vi "Dialog_debug (SubVI).vi"() -> ()   [LabVIEW 2017]
doc: "Use this template to create a dialog box with event handling."
uses:
  Control_EU/UNDT_ClusterPackRevers (Type).ctl
  Global_SNK3_HF.vi
panel:
  in  "Tab Control":enum32{"UNDT_Cl 1", "Page 2"}(tab)
  out "UNDT_Cl0":T1={"PacketCounter"=998360, "Gain Coeff"=0.0, "SamplingInterval"=2e-08, "Lose Packet"=8, "EncodersParam2"=0, "EncodersParam1"=0, "Reserve 1"=0, "Mux TX/RX"=0, "ScanDelay"=0, "CRC 8"=86, "ScanDuration"=500, "N chanel"=0, "GlobalTime2"=63660000, "GlobalTime1"=11423, "N tick"=0, "Ncycle"=15329, "FrameFormatVersion"=1, "MagicWord"=305419896, "Overload"=FALSE} {"Gain Coeff" format="%_5e"; "Reserve 1" format="%02x"; "Mux TX/RX" format="%02x"; "ScanDelay" format="%02x"; "SamplingInterval" format="%_3e"; "Lose Packet" format="%08x"; "EncodersParam2" format="%016x"; "EncodersParam1" format="%016x"; "CRC 8" format="%02x"; "N chanel" format="%02x"; "N tick" format="%02x"; "FrameFormatVersion" format="%02x"; "MagicWord" format="%.0x"}
  out "UNDT_Cl1":T1={"PacketCounter"=998360, "Gain Coeff"=0.0, "SamplingInterval"=2e-08, "Lose Packet"=8, "EncodersParam2"=0, "EncodersParam1"=0, "Reserve 1"=0, "Mux TX/RX"=0, "ScanDelay"=0, "CRC 8"=86, "ScanDuration"=500, "N chanel"=0, "GlobalTime2"=63660000, "GlobalTime1"=11423, "N tick"=0, "Ncycle"=15329, "FrameFormatVersion"=1, "MagicWord"=305419896, "Overload"=FALSE} {"Gain Coeff" format="%_5e"; "Reserve 1" format="%02x"; "Mux TX/RX" format="%02x"; "ScanDelay" format="%02x"; "SamplingInterval" format="%_3e"; "Lose Packet" format="%08x"; "EncodersParam2" format="%016x"; "EncodersParam1" format="%016x"; "CRC 8" format="%02x"; "N chanel" format="%02x"; "N tick" format="%02x"; "FrameFormatVersion" format="%02x"; "MagicWord" format="%.0x"}
  out "UDP0_iter_count":i32=7055
  out "UDP0_timeout":i32=1000
  out "UDP0_port":u16=1555
  out "UDP0_address":u32=3232235999 format="%x"
  out "UDP0_AscanLostPack":u32
  out "UDP0_offset":i32
  out "UDP0_Reserv":u8
  out "UDP0_length":i32=2052
  out "UDP0_packet_nuber":u32=1995311
  out "UDP0_packet_size":u16=652
  out "UDP0_LostPack":u32 caption="UDP0__lost_pack"
  out "UDP0_CRC8_bad":u32
  out "UDP0_PackEnd_bad":u32
  in  "stop":bool
  out "TblParam0":sgl[][](array[numeric])
  out "TblParam1":sgl[][](array[numeric])
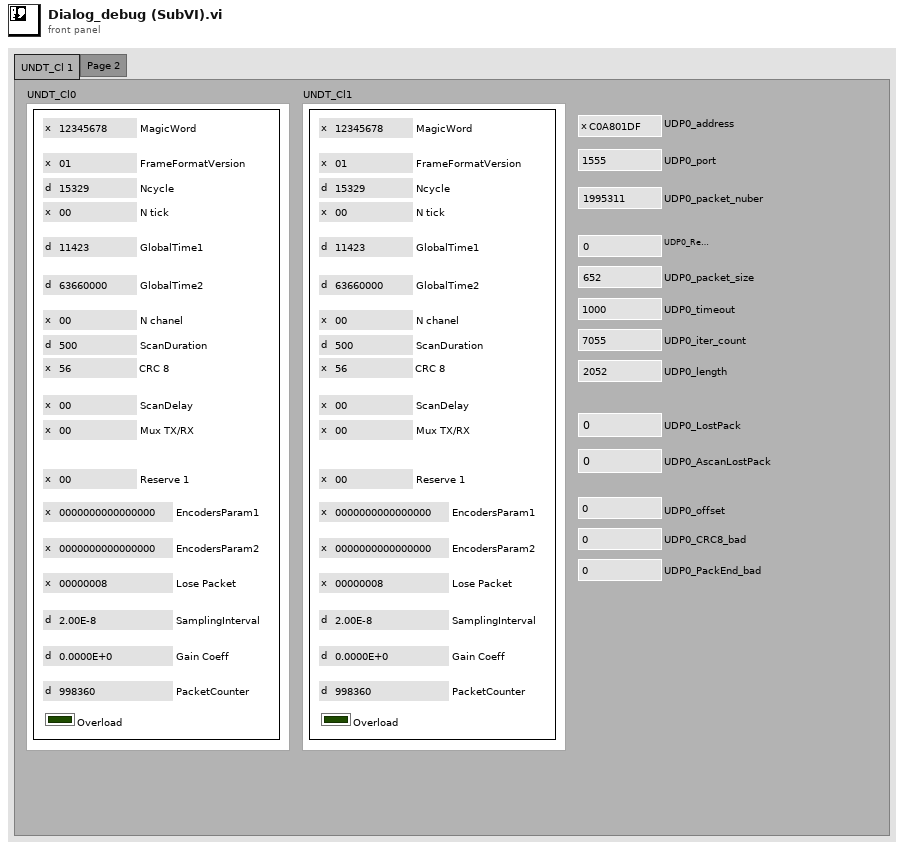
[diagram p1: front panel]
types:
  T1 = typedef "UNDT_ClusterPackRevers (Type).ctl" = cluster{"PacketCounter":u32, "Gain Coeff":sgl, "SamplingInterval":sgl, "Lose Packet":u32, "EncodersParam2":u64, "EncodersParam1":u64, "Reserve 1":u8, "Mux TX/RX":u8, "ScanDelay":u16, "CRC 8":u8, "ScanDuration":u16, "N chanel":u8, "GlobalTime2":u32, "GlobalTime1":u32, "N tick":u8, "Ncycle":u16, "FrameFormatVersion":u8, "MagicWord":u32, "Overload":bool}
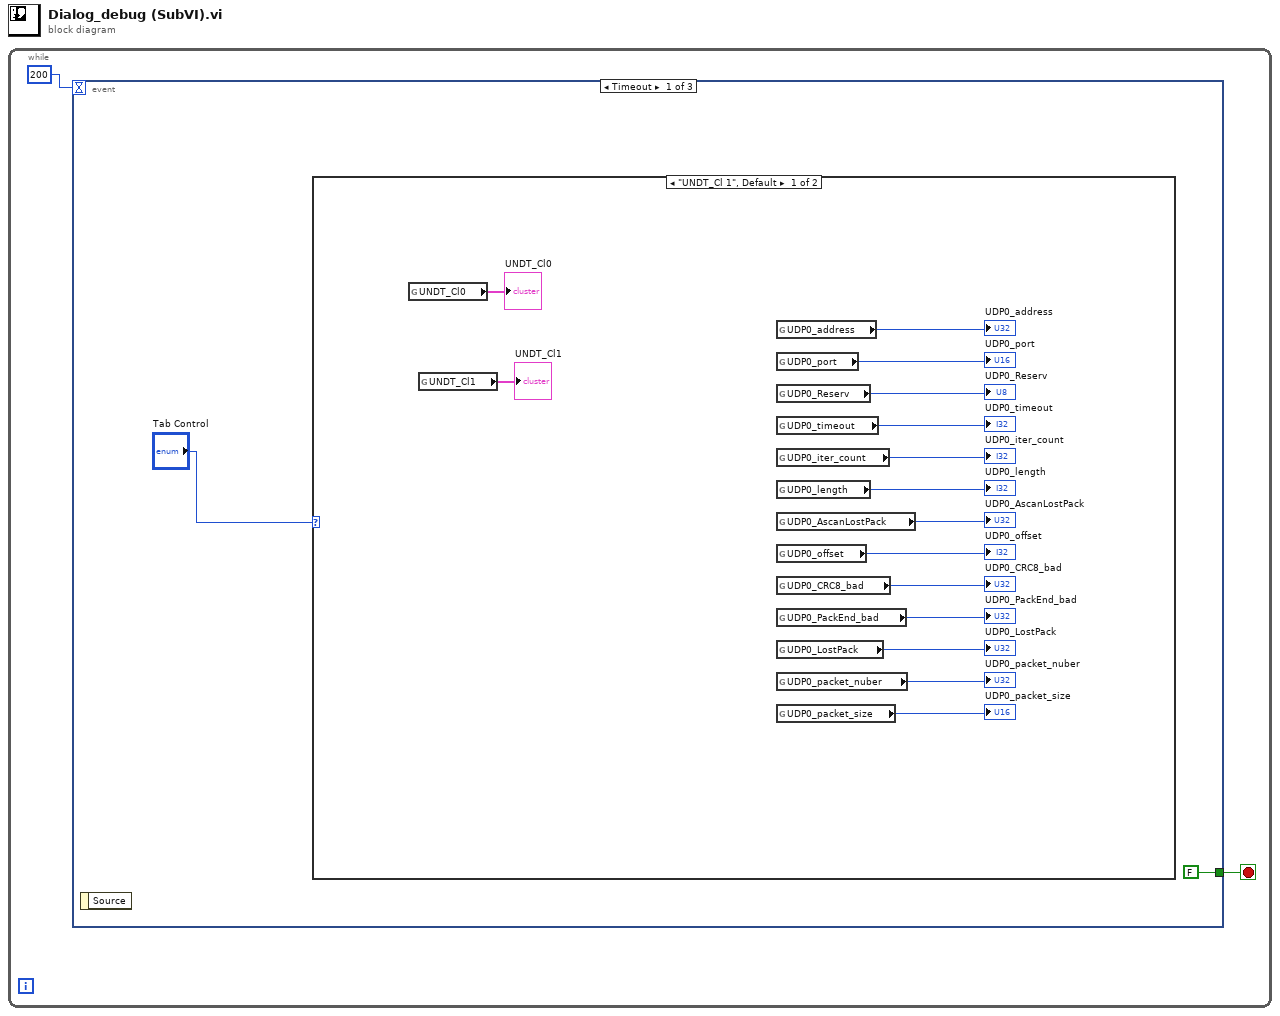
[diagram p0: block diagram]
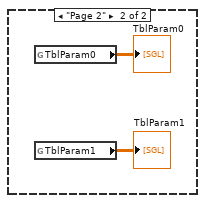
[diagram p2: hidden frame]
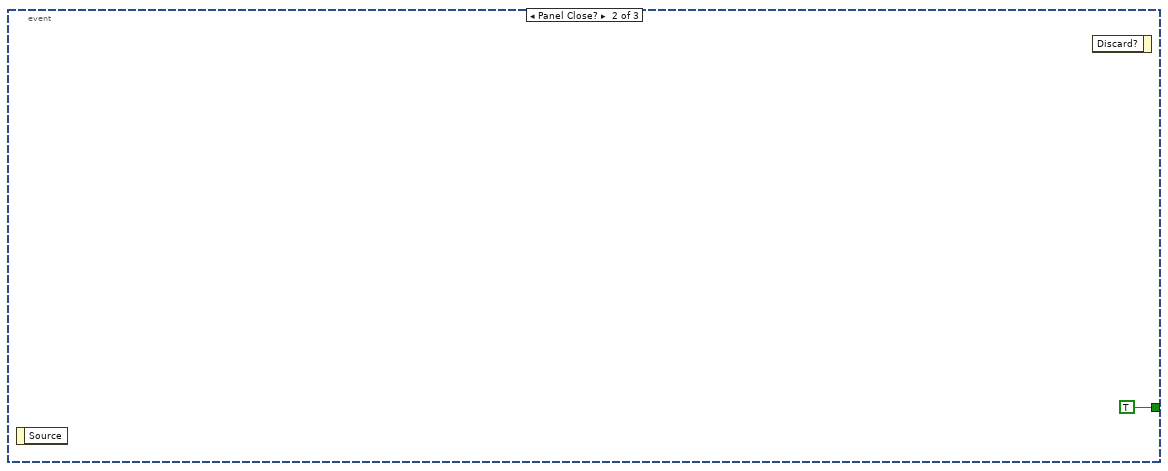
[diagram p3: hidden frame]
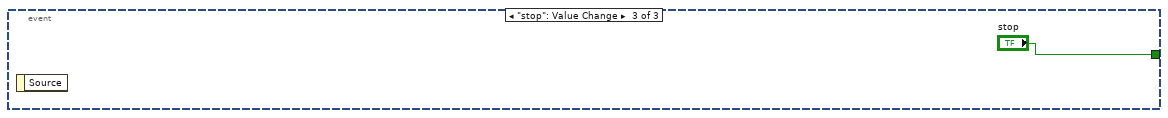
[diagram p4: hidden frame]
diagram:
  n1 = while {
    stop <- w2 stop-if-true
    n2 = event shown="[0] Timeout" {
      selector: _ -> [_ _ _]
      dyn-events: _ -> [_ _ _]
      timeout: 200 -> [_ _ _]
      tunnel: [FALSE ("stop") TRUE ("Stop?") "stop"] -> w2
      event Timeout {
        n3 = event-data() -> ()  [unwired: 1 in, 1 out]
        n4 = case shown="\"UNDT_Cl 1\", Default" "Tab Control" {
          frame "UNDT_Cl 1", Default {
            n5 = global read "Global_SNK3_HF.vi" "UNDT_Cl0"() -> (→"UNDT_Cl0":T1)
            n6 = global read "Global_SNK3_HF.vi" "UNDT_Cl1"() -> (→"UNDT_Cl1":T1)
            n7 = global read "Global_SNK3_HF.vi" "UDP0_address"() -> (→"UDP0_address":u32)
            n8 = global read "Global_SNK3_HF.vi" "UDP0_port"() -> (→"UDP0_port":u16)
            n9 = global read "Global_SNK3_HF.vi" "UDP0_Reserv"() -> (→"UDP0_Reserv":u8)
            n10 = global read "Global_SNK3_HF.vi" "UDP0_timeout"() -> (→"UDP0_timeout":i32)
            n11 = global read "Global_SNK3_HF.vi" "UDP0_iter_count"() -> (→"UDP0_iter_count":i32)
            n12 = global read "Global_SNK3_HF.vi" "UDP0_length"() -> (→"UDP0_length":i32)
            n13 = global read "Global_SNK3_HF.vi" "UDP0_AscanLostPack"() -> (→"UDP0_AscanLostPack":u32)
            n14 = global read "Global_SNK3_HF.vi" "UDP0_offset"() -> (→"UDP0_offset":i32)
            n15 = global read "Global_SNK3_HF.vi" "UDP0_CRC8_bad"() -> (→"UDP0_CRC8_bad":u32)
            n16 = global read "Global_SNK3_HF.vi" "UDP0_PackEnd_bad"() -> (→"UDP0_PackEnd_bad":u32)
            n17 = global read "Global_SNK3_HF.vi" "UDP0_LostPack"() -> (→"UDP0_LostPack":u32)
            n18 = global read "Global_SNK3_HF.vi" "UDP0_packet_nuber"() -> (→"UDP0_packet_nuber":u32)
            n19 = global read "Global_SNK3_HF.vi" "UDP0_packet_size"() -> (→"UDP0_packet_size":u16)
          }
          frame "Page 2" {
            n20 = global read "Global_SNK3_HF.vi" "TblParam0"() -> (→"TblParam0":sgl[][])
            n21 = global read "Global_SNK3_HF.vi" "TblParam1"() -> (→"TblParam1":sgl[][])
          }
        }
      }
      event Panel Close? {
        n22 = event-data() -> ()  [unwired: 1 in, 1 out]
        n23 = event-data() -> ()  [unwired: 2 in, 1 out]
      }
      event "stop": Value Change {
        n24 = event-data() -> ()  [unwired: 1 in, 1 out]
      }
    }
  }
